vi "Motor.vi"() -> ()   [LabVIEW 2023]
uses:
  <vilib>/Instr/_visa.llb/VISA Configure Serial Port (Instr).vi
panel:
  in  "Time intervals":u32=500
  in  "Final Position":dbl=1600.0
  in  "Scan":bool
  in  "Step size":dbl=250.0
  in  "Start/End Position":u16(ring) caption="Ring" items=["Start position", "End position"]
  in  "GO":bool
  in  "Pulse PIN (Z - Axis)":string="12"
  in  "Pulse PIN (Y - Axis)":string="11"
  in  "Pulse PIN (X - Axis)":string="10"
  in  "Select Axis":u16(ring) caption="Ring" items=["X - Axis", "Y - Axis", "Z - Axis"]
  in  "STEP":dbl(slide)=500.0 scale=250.0..1500.0
  in  "Movement direction":u16(ring) caption="Ring" items=["Backward", "Forward"]
  in  "Enable PIN":string="08"
  in  "Direction PIN":string="09" caption="Dirrection PIN"
  in  "SPEED":dbl(slide)=500.0 scale=250.0..1500.0
  in  "Stop Process":bool
  in  "MOVE":bool
  in  "VISA Port":refnum<visa-resource-name>="COM3"
  # "Arduino Uno Pins"
  # "Scan Option"
  # "Under development"
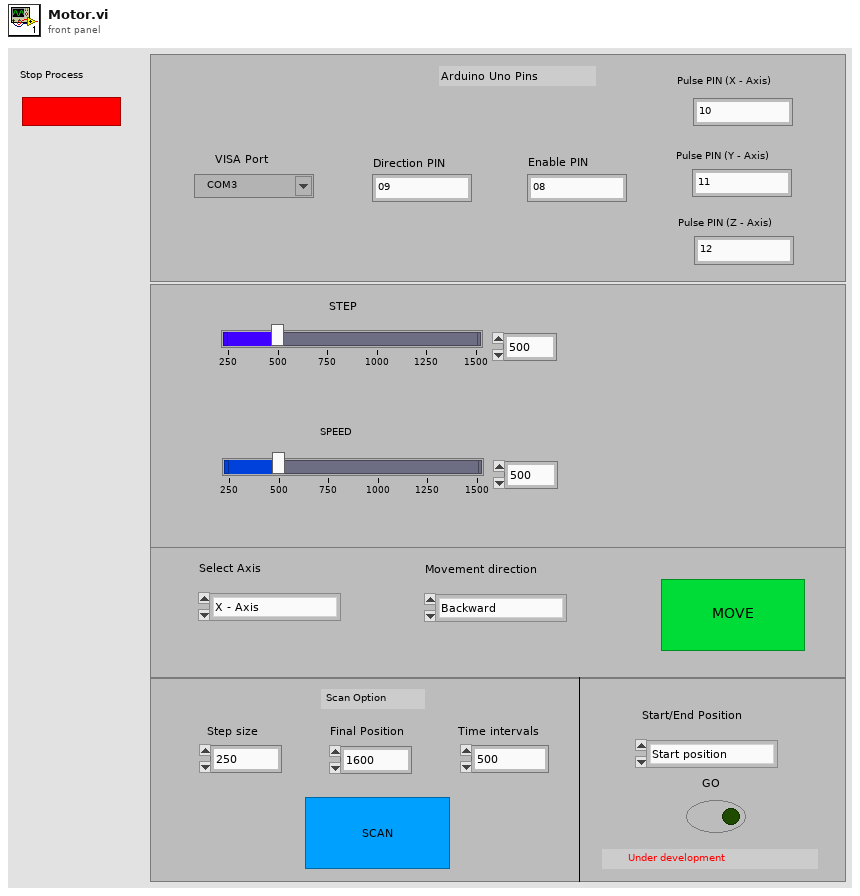
[diagram p1: front panel]
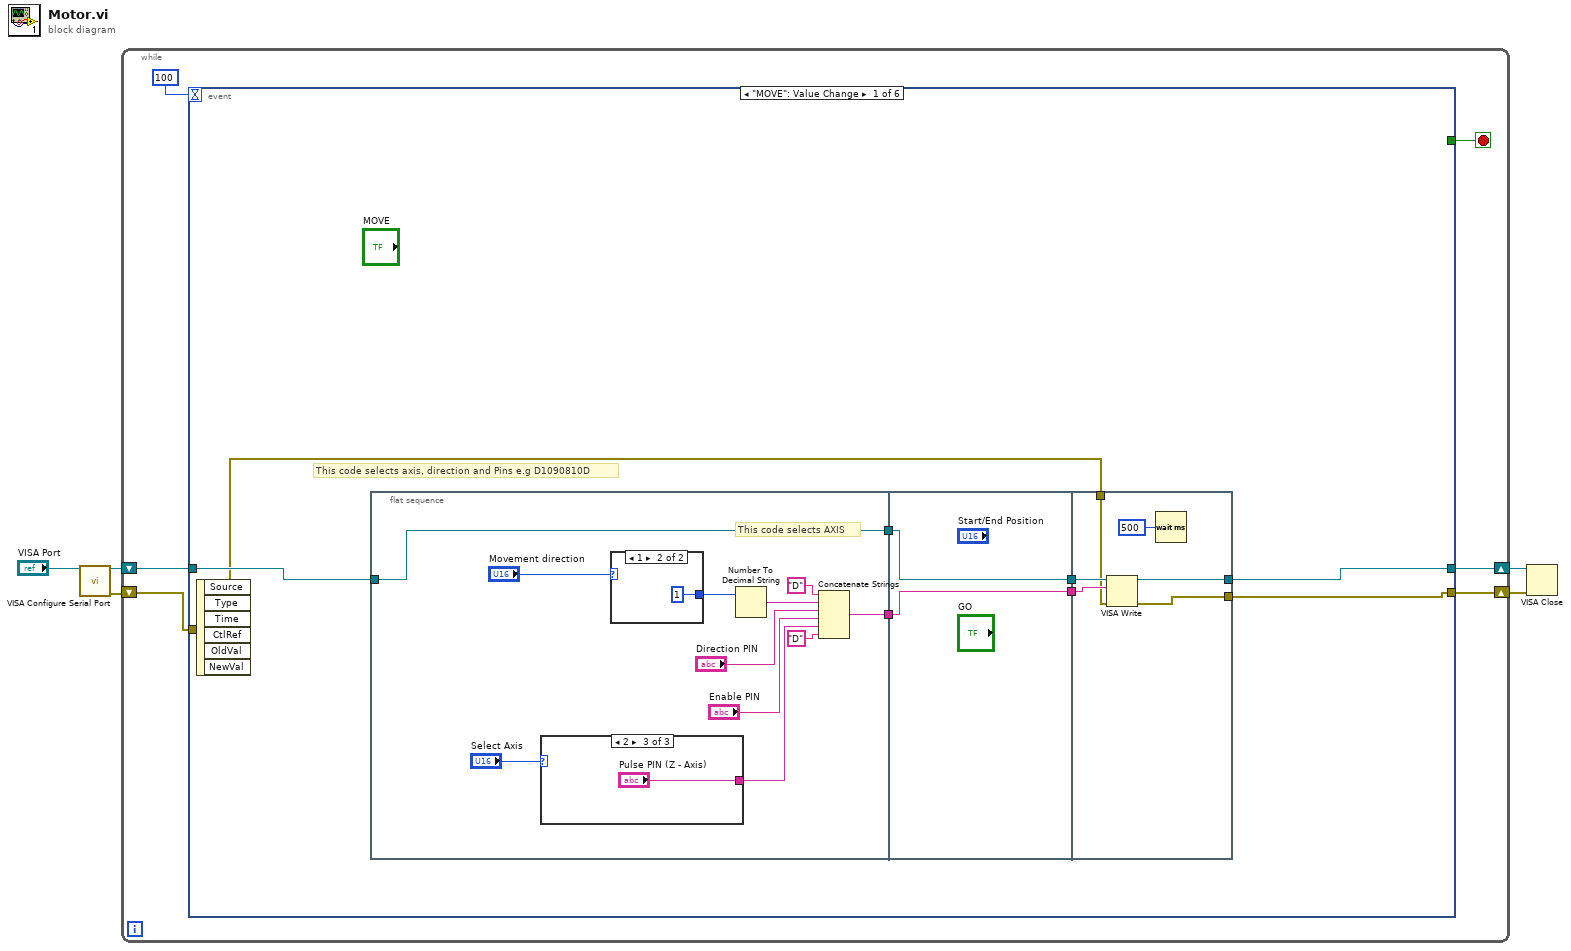
[diagram p0: block diagram]
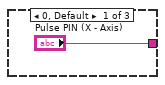
[diagram p2: hidden frame]
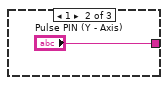
[diagram p3: hidden frame]
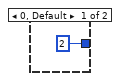
[diagram p4: hidden frame]
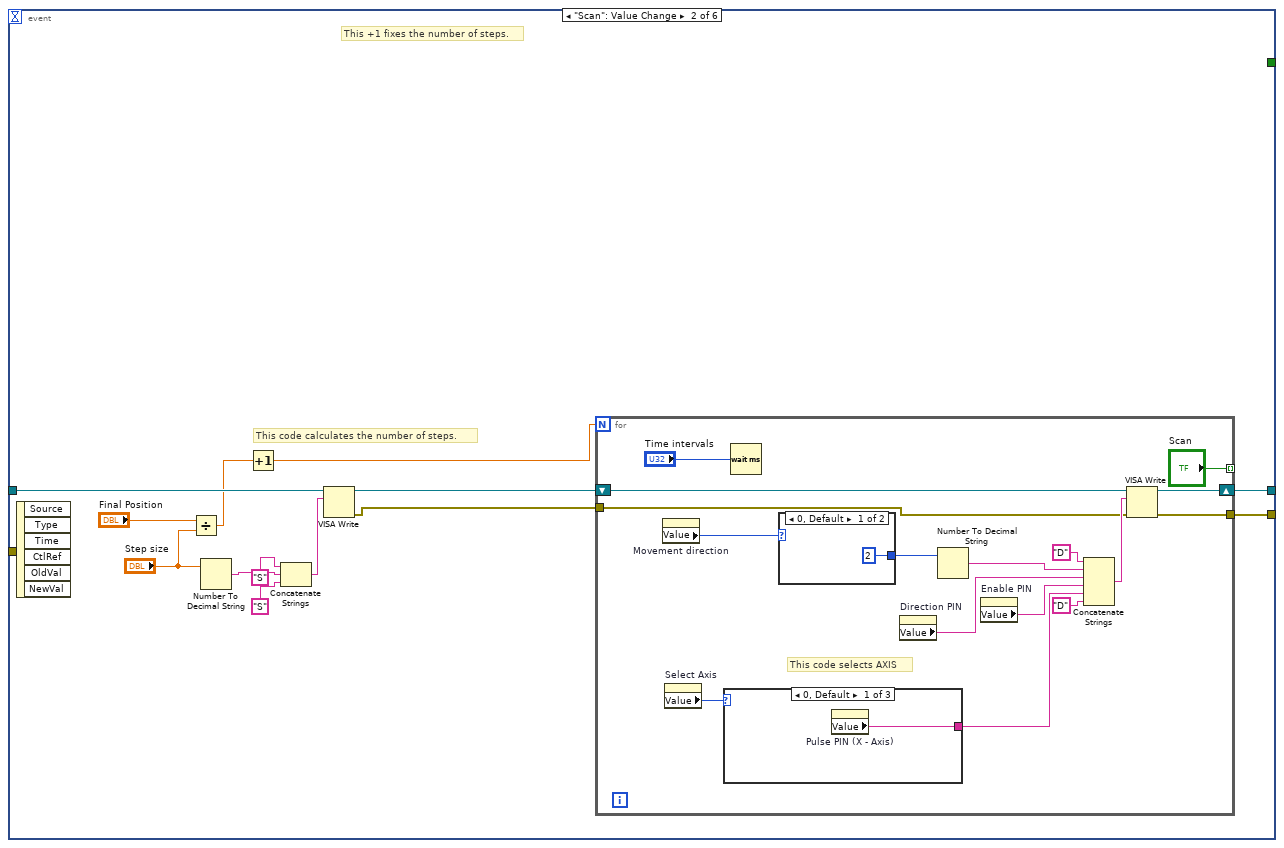
[diagram p5: hidden frame]
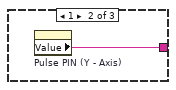
[diagram p6: hidden frame]
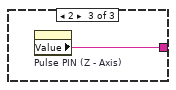
[diagram p7: hidden frame]
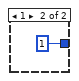
[diagram p8: hidden frame]
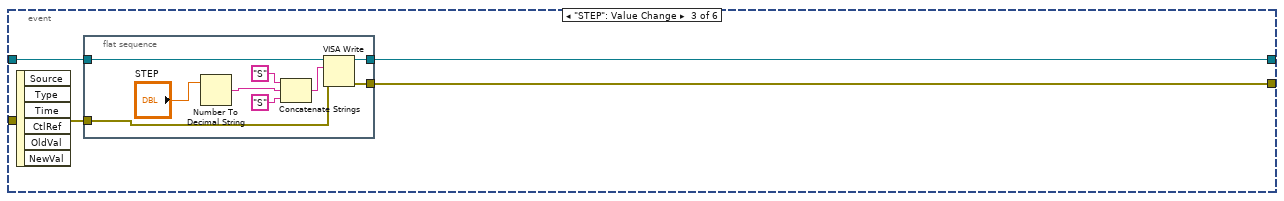
[diagram p9: hidden frame]
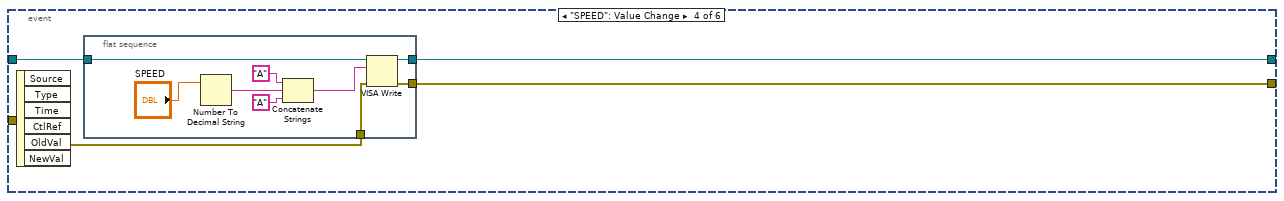
[diagram p10: hidden frame]
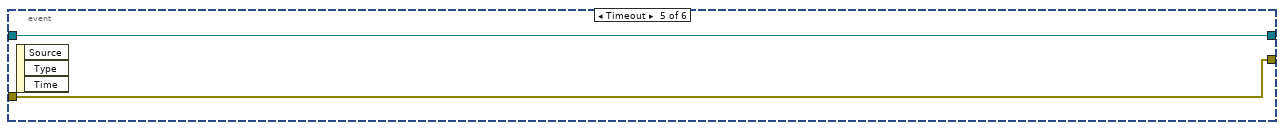
[diagram p11: hidden frame]
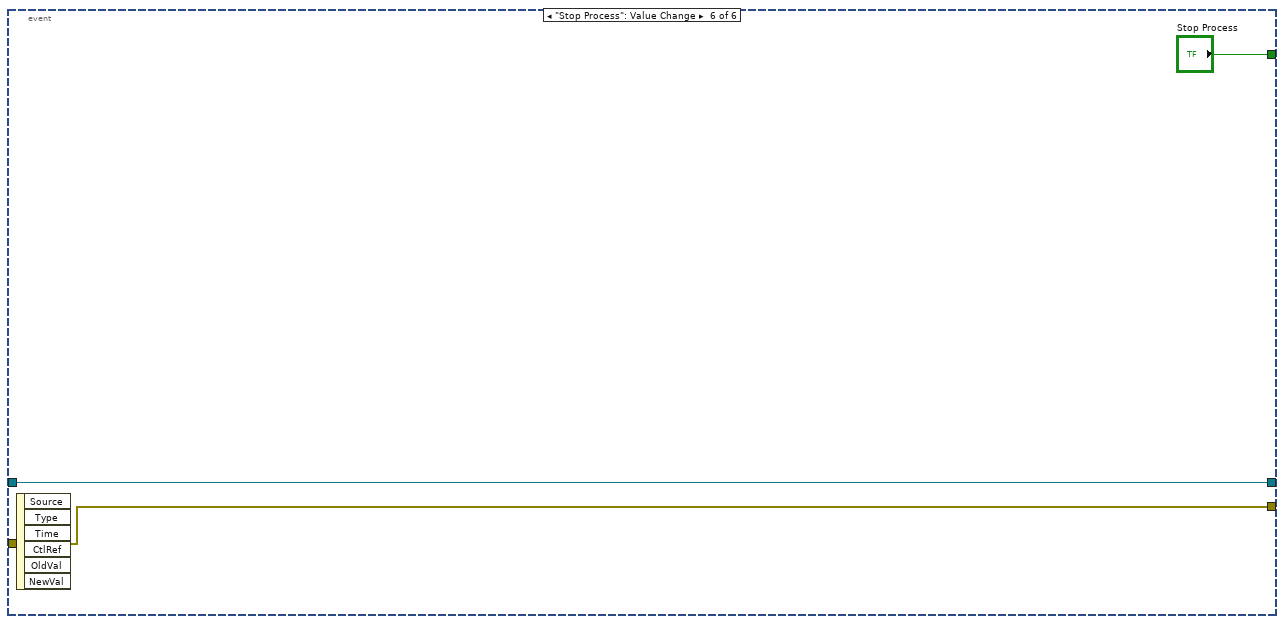
[diagram p12: hidden frame]
diagram:
  n1 = call-poly "VISA Configure Serial Port"("VISA resource name"="VISA Port") -> ("VISA resource name out"=w4:refnum<visa-resource-name>, "error out"=w2:errorcluster)  [unwired: 13 in]
  n2 = while {
    shift-right: [w10] -> w3
    shift-left: w4 -> [w11]
    shift-right: [w6] -> w1
    shift-left: w2 -> [w7]
    stop <- w9 stop-if-true
    n3 = event shown="[0] \"MOVE\": Value Change" {
      selector: _ -> [_ _ _ _ _ _]
      dyn-events: _ -> [_ _ _ _ _ _]
      timeout: 100 -> [_ _ _ _ _ _]
      tunnel: w11 -> [w18 w50 w80 w94 w105 w107]
      tunnel: [w19 w56 w81 w93 w105 w107] -> w10
      tunnel: [_ _ _ _ _ "Stop Process"] -> w9
      tunnel: w7 -> [w12 _ w79 w92 w104 w106]
      tunnel: [w13 w44 w78 w91 w104 w106] -> w6
      event "MOVE": Value Change {
        # "This code selects axis, direction and Pins e.g D1090810D"
        n4 = event-data() -> ()  [unwired: 1 in, 6 out]
        n5 = flat-sequence {
          tunnel: [w23] -> w17
          tunnel: w18 -> [w22]
          tunnel: [w22] -> w15
          tunnel: w17 -> [w37]
          tunnel: [w37] -> w16
          tunnel: w15 -> [w36]
          tunnel: [w36] -> w14
          tunnel: [w42] -> w19
          tunnel: w16 -> [w41]
          tunnel: w14 -> [w43]
          tunnel: [w39] -> w13
          tunnel: w12 -> [w38]
          frame #0 {
            # "This code selects AXIS"
            n6 = case shown="2" "Select Axis" {
              tunnel: ["Pulse PIN (X - Axis)" "Pulse PIN (Y - Axis)" "Pulse PIN (Z - Axis)"] -> w21
              frame 0, Default {
              }
              frame 1 {
              }
              frame 2 {
              }
            }
            n7 = case shown="1" "Movement direction" {
              tunnel: [2 1] -> w25
              frame 0, Default {
              }
              frame 1 {
              }
            }
            n8 = Number To Decimal String(number=w25) -> (decimal integer string=w30:string)  [unwired: 1 in]
            n9 = Concatenate Strings("D" ("string"), w30, "Direction PIN", "Enable PIN", w21, "D" ("string")) -> (w23:string)
          }
          frame #1 {
          }
          frame #2 {
            n10 = VISA Write(VISA resource name=w43, write buffer=w41, error in (no error)=w38) -> (VISA resource name out=w42:refnum<visa-resource-name>, error out=w39:errorcluster)  [unwired: 1 out]
            n11 = Wait (ms)(milliseconds to wait=u32 500) -> ()  [unwired: 1 out]
          }
        }
      }
      event "Scan": Value Change {
        # "This +1 fixes the number of steps."
        # "This code calculates the number of steps."
        n12 = event-data() -> ()  [unwired: 1 in, 6 out]
        n13 = Divide(x="Final Position", y="Step size") -> (x/y=w46:dbl)
        n14 = Number To Decimal String(number="Step size") -> (decimal integer string=w54:string)  [unwired: 1 in]
        n15 = Increment(x=w46) -> (x+1=w47:dbl)
        n16 = Concatenate Strings("S", w54, "S") -> (w55:string)
        n17 = VISA Write(VISA resource name=w50, write buffer=w55) -> (VISA resource name out=w51:refnum<visa-resource-name>, error out=w45:errorcluster)  [unwired: 1 in, 1 out]
        n18 = for {
          N: w47 -> [_]
          shift-right: [w62] -> w56
          shift-left: w51 -> [w61]
          tunnel: ["Scan"] -> _ mode=indexing
          tunnel: w45 -> [w58]
          tunnel: [w57] -> w44
          # "This code selects AXIS"
          n19 = property on="Movement direction" class="Ring (strict)"() -> ("Value"=w64:u16)  [unwired: 2 in, 2 out]
          n20 = property on="Select Axis" class="Ring (strict)"() -> ("Value"=w65:u16)  [unwired: 2 in, 2 out]
          n21 = case shown="0, Default" w65 {
            tunnel: [w73 w74 w75] -> w68
            frame 0, Default {
              n22 = property on="Pulse PIN (X - Axis)" class="Str"() -> ("Value"=w73:string)  [unwired: 2 in, 2 out]
            }
            frame 1 {
              n23 = property on="Pulse PIN (Y - Axis)" class="Str"() -> ("Value"=w74:string)  [unwired: 2 in, 2 out]
            }
            frame 2 {
              n24 = property on="Pulse PIN (Z - Axis)" class="Str"() -> ("Value"=w75:string)  [unwired: 2 in, 2 out]
            }
          }
          n25 = Wait (ms)(milliseconds to wait="Time intervals") -> ()  [unwired: 1 out]
          n26 = case shown="0, Default" w64 {
            tunnel: [2 1] -> w69
            frame 0, Default {
            }
            frame 1 {
            }
          }
          n27 = property on="Direction PIN" class="Str"() -> ("Value"=w67:string)  [unwired: 2 in, 2 out]
          n28 = Number To Decimal String(number=w69) -> (decimal integer string=w72:string)  [unwired: 1 in]
          n29 = property on="Enable PIN" class="Str"() -> ("Value"=w66:string)  [unwired: 2 in, 2 out]
          n30 = Concatenate Strings("D" ("string"), w72, w67, w66, w68, "D" ("string")) -> (w63:string)
          n31 = VISA Write(VISA resource name=w61, write buffer=w63, error in (no error)=w58) -> (VISA resource name out=w62:refnum<visa-resource-name>, error out=w57:errorcluster)  [unwired: 1 out]
        }
      }
      event "STEP": Value Change {
        n32 = event-data() -> ()  [unwired: 1 in, 6 out]
        n33 = flat-sequence {
          tunnel: [w87] -> w81
          tunnel: w80 -> [w86]
          tunnel: [w83] -> w78
          tunnel: w79 -> [w82]
          frame #0 {
            n34 = Number To Decimal String(number="STEP") -> (decimal integer string=w88:string)  [unwired: 1 in]
            n35 = Concatenate Strings("S", w88, "S") -> (w85:string)
            n36 = VISA Write(VISA resource name=w86, write buffer=w85, error in (no error)=w82) -> (VISA resource name out=w87:refnum<visa-resource-name>, error out=w83:errorcluster)  [unwired: 1 out]
          }
        }
      }
      event "SPEED": Value Change {
        n37 = event-data() -> ()  [unwired: 1 in, 6 out]
        n38 = flat-sequence {
          tunnel: w94 -> [w99]
          tunnel: [w98] -> w93
          tunnel: [w96] -> w91
          tunnel: w92 -> [w95]
          frame #0 {
            n39 = Number To Decimal String(number="SPEED") -> (decimal integer string=w101:string)  [unwired: 1 in]
            n40 = Concatenate Strings("A", w101, "A") -> (w100:string)
            n41 = VISA Write(VISA resource name=w99, write buffer=w100, error in (no error)=w95) -> (VISA resource name out=w98:refnum<visa-resource-name>, error out=w96:errorcluster)  [unwired: 1 out]
          }
        }
      }
      event Timeout {
        n42 = event-data() -> ()  [unwired: 1 in, 3 out]
      }
      event "Stop Process": Value Change {
        n43 = event-data() -> ()  [unwired: 1 in, 6 out]
      }
    }
  }
  n44 = VISA Close(VISA resource name=w3, error in (no error)=w1) -> ()  [unwired: 1 out]
